vi "Encode Command.vi"(0 "Function":string(combo), 1 "Address":string="X", 9 "Data":string) -> (4 "Command out":string)   [LabVIEW 2020, in "UART.lvlib"]
uses:
  UART/UART.lvlib
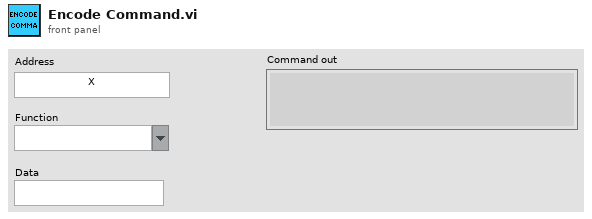
[diagram p1: front panel]
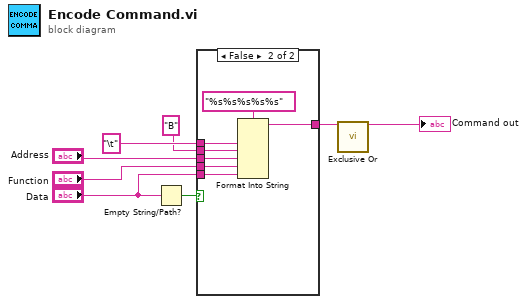
[diagram p0: block diagram]
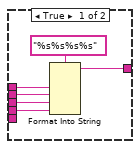
[diagram p2: hidden frame]
diagram:
  n1 = Empty String/Path?(string/path="Data") -> (empty?=w4:bool)
  n2 = case shown="False" w4 {
    tunnel: "\t" -> [w14 w21]
    tunnel: "B" -> [w13 w20]
    tunnel: "Address" -> [w12 w19]
    tunnel: "Function" -> [w11 w18]
    tunnel: "Data" -> [_ w17]
    tunnel: [w9 w15] -> w2
    frame True {
      n3 = Format Into String(format string="%s%s%s%s", w14, w13, w12, w11) -> (resulting string=w9:string)  [unwired: 2 in, 1 out]
    }
    frame False {
      n4 = Format Into String(format string="%s%s%s%s%s", w21, w20, w19, w18, w17) -> (resulting string=w15:string)  [unwired: 2 in, 1 out]
    }
  }
  n5 = call "Exclusive Or.vi"("String"=w2) -> ("String OutPut"=→"Command out":string)  [unwired: 12 in, 2 out]
